vi "Message decoding.vi"(8 "error in (no error)":errorcluster, 10 "Message":string, 11 "TCP Text Listener in":refnum<class "TCP Text Listener.lvclass">) -> (0 "error out":errorcluster, 2 "Message decoded":T1, 3 "TCP Text Listener out":refnum<class "TCP Text Listener.lvclass">)   [LabVIEW 2026, in "TALOS.lvlib" / "TCP Text Listener.lvlib" / "TCP Text Listener.lvclass"]
uses:
  TCP Text Listener.lvclass
  TCP Writer/TCP Writer/TCP Message Internal Composition.ctl
  <vilib>/Utility/error.llb/Trim Whitespace (string).vi
  <vilib>/AdvancedString/Delimited String to 1D String Array (string).vi
  <vilib>/Utility/error.llb/Trim Whitespace One-Sided.vi
  Support VIs/Global Constants.vi
  TALOS.lvlib
  TCP Writer/TCP Writer/TCP Writer.lvclass
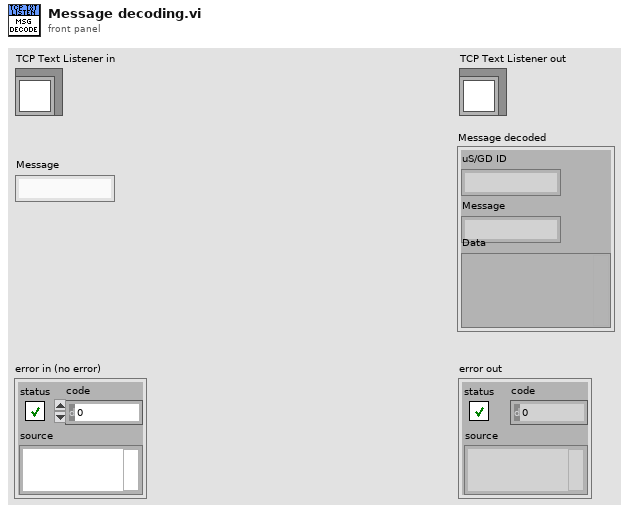
[diagram p1: front panel]
types:
  T1 = typedef "TALOS.lvlib/TCP Writer.lvlib/TCP Writer.lvclass/TCP Message Internal Composition.ctl" = cluster{"uS/GD ID":string, "Message":string, "Data":variant}
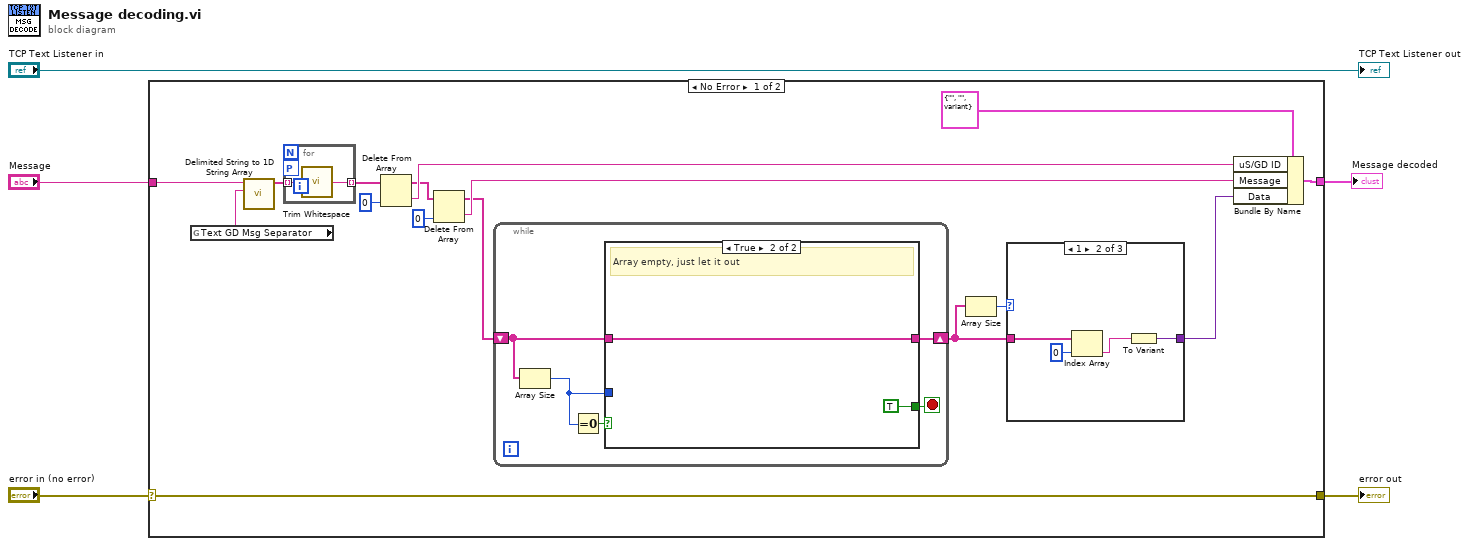
[diagram p0: block diagram]
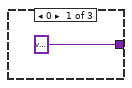
[diagram p2: hidden frame]
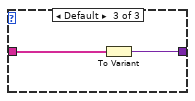
[diagram p3: hidden frame]
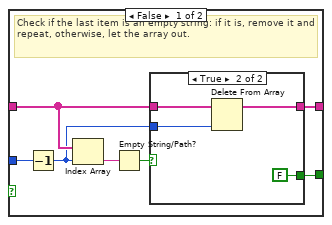
[diagram p4: hidden frame]
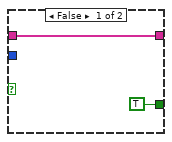
[diagram p5: hidden frame]
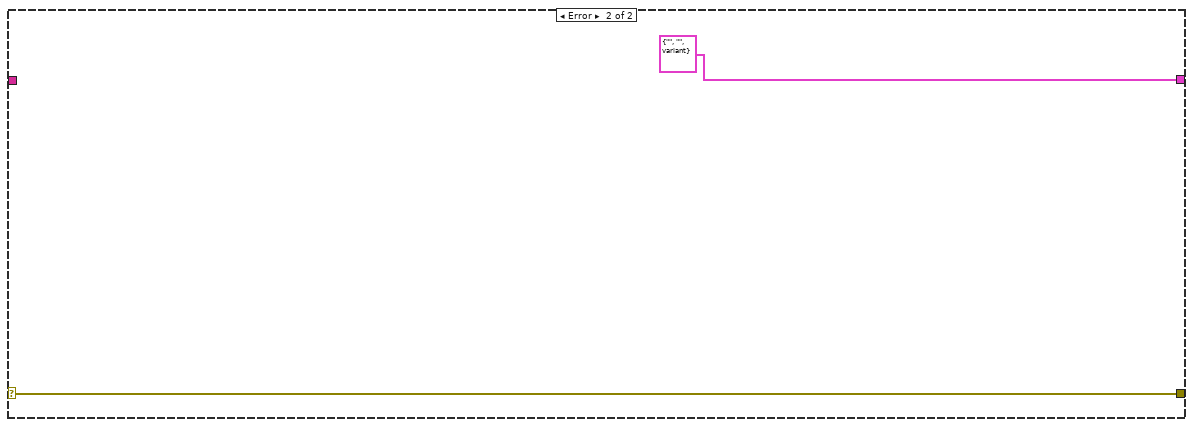
[diagram p6: hidden frame]
diagram:
  n1 = case shown="No Error" "error in (no error)" {
    selector: "error in (no error)" -> [w9 w51]
    tunnel: "Message" -> [w13 _]
    tunnel: [w10 T1 {"uS/GD ID"="", "Message"="", "Data"=variant} ("TCP Message Internal Composition")] -> w3
    tunnel: [w9 w51] -> w1
    frame No Error {
      n2 = global read "Global Constants.vi" "Text GD Msg Separator"() -> (w12:string)
      n3 = call-poly <vilib>:"Delimited String to 1D String Array.vi"("delimiter"=w12, "delimited string"=w13) -> ("string array"=w21:string[])  [unwired: 9 in]
      n4 = for {
        tunnel: w21 -> [w50] mode=indexing
        tunnel: [w49] -> w20 mode=indexing
        workers-P: _ -> [_]
        n5 = call-poly <vilib>:"Trim Whitespace.vi"("string"=w50) -> ("trimmed string"=w49:string)  [unwired: 1 in]
      }
      n6 = Delete From Array(array=w20, index=0) -> (deleted portion=w18:string, array with subset deleted=w17:string[])  [unwired: 1 in]
      n7 = Delete From Array(array=w17, index=0) -> (deleted portion=w15:string, array with subset deleted=w14:string[])  [unwired: 1 in]
      n8 = while {
        shift-right: [w30] -> w7
        shift-left: w14 -> [w31]
        stop <- w29 stop-if-true
        n9 = Array Size(array=w31) -> (size(s)=w33:i32)
        n10 = Equal To 0?(x=w33) -> (x = 0?=w32:bool)
        n11 = case shown="True" w32 {
          tunnel: w33 -> [w40 _]
          tunnel: w31 -> [w36 w48]
          tunnel: [w37 w48] -> w30
          tunnel: [w35 TRUE] -> w29
          frame False {
            # "Check if the last item is an empty string: if it is, remove it and repeat, otherwise, let the array out."
            n12 = Decrement(x=w40) -> (x-1=w34:i32)
            n13 = Index Array(array=w36, index=w34) -> (element=w39:string)
            n14 = Empty String/Path?(string/path=w39) -> (empty?=w38:bool)
            n15 = case shown="True" w38 {
              tunnel: [w42 w44] -> w37
              tunnel: w36 -> [w42 w46]
              tunnel: [TRUE FALSE] -> w35
              tunnel: w34 -> [_ w45]
              frame False {
              }
              frame True {
                n16 = Delete From Array(array=w46, index=w45) -> (array with subset deleted=w44:string[])  [unwired: 1 in, 1 out]
              }
            }
          }
          frame True {
            # "Array empty, just let it out"
          }
        }
      }
      n17 = Array Size(array=w7) -> (size(s)=w8:i32)
      n18 = case shown="1" w8 {
        tunnel: w7 -> [_ w26 w28]
        tunnel: [variant w23 w27] -> w6
        frame 0 {
        }
        frame 1 {
          n19 = Index Array(array=w26, index=0) -> (element=w24:string)
          n20 = To Variant(anything=w24) -> (Variant=w23:variant)
        }
        frame Default {
          n21 = To Variant(anything=w28) -> (Variant=w27:variant)
        }
      }
      n22 = Bundle By Name(cluster=T1 {"uS/GD ID"="", "Message"="", "Data"=variant} ("TCP Message Internal Composition"), "uS/GD ID"=w18, "Message"=w15, "Data"=w6) -> (w10:T1)
    }
    frame Error {
    }
  }
  "error out" <- w1
  "Message decoded" <- w3
  "TCP Text Listener out" <- "TCP Text Listener in"
